vi "input.vi"(8 "error in":errorcluster, 10 "data table in":T5, 11 "SystemLin Tag Module runtime in":refnum<class "SystemLink runtime.lvclass">) -> (0 "error out":errorcluster, 2 "data table out":T5, 3 "SystemLin Tag Module runtime out":refnum<class "SystemLink runtime.lvclass">)   [LabVIEW 2015, in "SystemLink runtime.lvclass"]
doc: "Provides an interface for reading data from a module at runtime. While this interface performs no operations, a child should provide an override which may read from any open sessions, references, or interfaces."
uses:
  SystemLink runtime.lvclass
  <vilib>/NI/Tag Bus/table/data table.ctl
  <vilib>/Skyline/Tag/Shared/typedefs/Tag Value Cluster.ctl
  <vilib>/Skyline/Tag/Shared/typedefs/DataType.ctl
  configuration/SysLink Mapping.ctl
  <vilib>/Skyline/Tag/Wrapper/Wrapper_class/NI Skyline Tag.lvclass
  <vilib>/NI/Tag Bus/tag/Data Type.ctl
  SystemLink runtime.lvclass/SystemLink runtime.ctl
  <vilib>/NI/Tag Bus/table/data polymorphs/write one/write Double.vi
  <vilib>/NI/Tag Bus/table/data polymorphs/write one/write Single.vi
  <vilib>/NI/Tag Bus/table/data polymorphs/write one/write String.vi
  <vilib>/NI/Tag Bus/table/data polymorphs/write one/write I32.vi
  <vilib>/NI/Tag Bus/table/data polymorphs/write one/write U64.vi
  <vilib>/NI/Tag Bus/table/data polymorphs/write one/write I16.vi
  <vilib>/NI/Tag Bus/table/data polymorphs/write one/write I8.vi
  <vilib>/NI/Tag Bus/table/data polymorphs/write one/write Boolean.vi
  <vilib>/NI/Tag Bus/table/data table.lvlib
  <vilib>/Skyline/Tag/Wrapper/Wrapper_class/Read Tag (I32).vi
  <vilib>/Skyline/Tag/Wrapper/Wrapper_class/Read Tag (DBL).vi
  <vilib>/Skyline/Tag/Wrapper/Wrapper_class/Read Tag (String).vi
  <vilib>/Skyline/Tag/Shared/NI Skyline Tag.lvlib
  <vilib>/NI/Tag Bus/tag/tag descriptor.lvclass
  configuration/SystemLink configuration.lvclass
panel:
  out "Inputs Array":refnum<class "NI Skyline Tag.lvclass">[](array[class])
  out "Input Map":T1[](array[typedef])
  out "tag clusters":T3[](array[typedef])
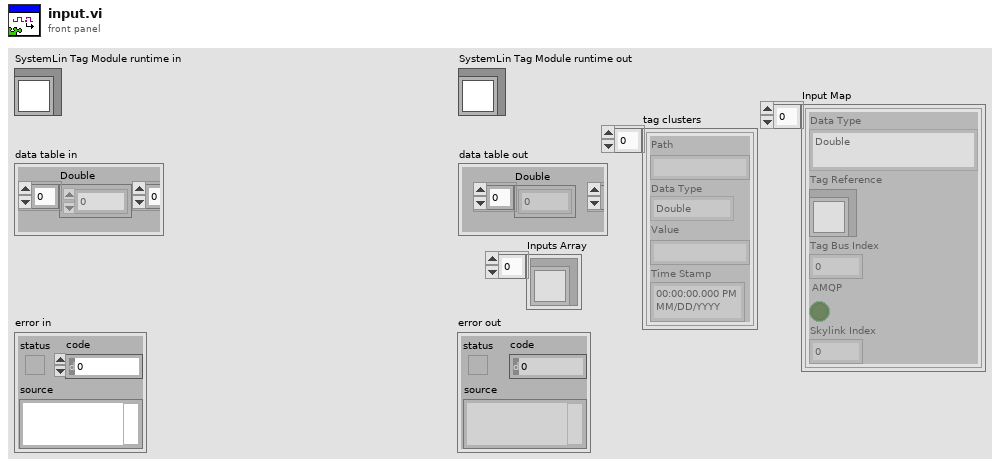
[diagram p1: front panel]
types:
  T1 = typedef "SystemLink configuration.lvclass/SysLink Mapping.ctl" = cluster{"Data Type":T2, "Tag Reference":refnum<class "NI Skyline Tag.lvclass">, "Tag Bus Index":i32, "AMQP":bool, "Skylink Index":i32}
  T2 = typedef "tag bus.lvlib/tag descriptor.lvclass/Data Type.ctl" = enum16{"Double", "Single", "I64", "I32", "I16", "I8", "U64", "U32", "U16", "U8", "Boolean", "String", "Array of Double", "Array of Single", "Array of I64", "Array of I32", "Array of I16", "Array of I8", "Array of U64", "Array of U32", "Array of U16", "Array of U8", "Array of Boolean", "Array of String"}
  T3 = typedef "NI Skyline Tag.lvlib/Tag Value Cluster.ctl" = cluster{"Path":string, "Data Type":T4, "Value":string, "Time Stamp":timestamp}
  T4 = typedef "NI Skyline Tag.lvlib/DataType.ctl" = enum32{"Double", "I32", "String", "Boolean", "U64", "Timestamp"}
  T5 = typedef "tag bus.lvlib/data table.lvlib/data table.ctl" = cluster{"Double":dbl[], "Single":sgl[], "I64":i64[], "I32":i32[], "I16":i16[], "I8":i8[], "U64":u64[], "U32":u32[], "U16":u16[], "U8":u8[], "Boolean":bool[], "String":string[], "Array of Double":cluster{"DBL Array":dbl[]}[], "Array of Single":cluster{"SGL Array":sgl[]}[], "Array of I64":cluster{"I64 Array":i64[]}[], "Array of I32":cluster{"I32 Array":i32[]}[], "Array of I16":cluster{"I16 Array":i16[]}[], "Array of I8":cluster{"I8 Array":i8[]}[], "Array of U64":cluster{"U64 Array":u64[]}[], "Array of U32":cluster{"U32 Array":u32[]}[], "Array of U16":cluster{"U16 Array":u16[]}[], "Array of U8":cluster{"U8 Array":u8[]}[], "Array of Boolean":cluster{"Boolean Array":bool[]}[], "Array of String":cluster{"String Array":string[]}[]}
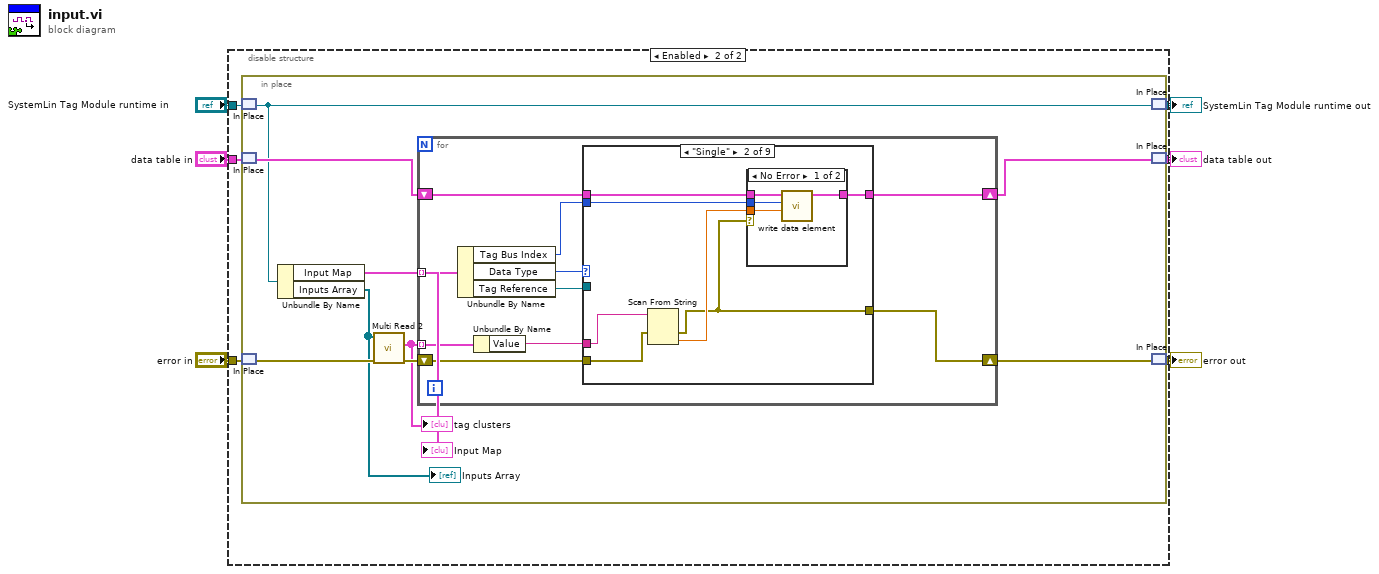
[diagram p0: block diagram]
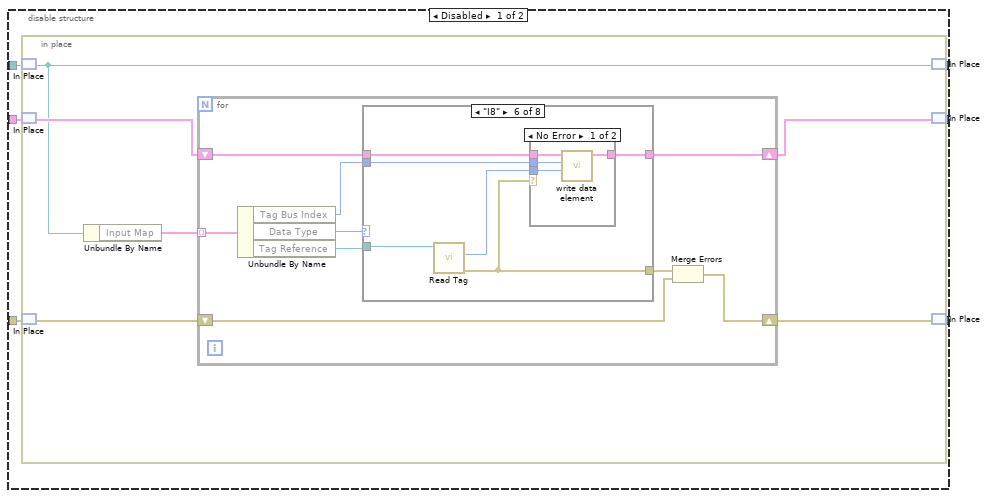
[diagram p2: hidden frame]
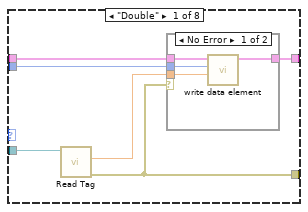
[diagram p3: hidden frame]
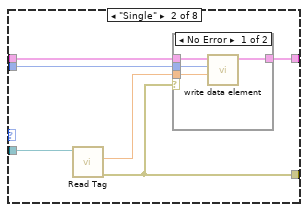
[diagram p5: hidden frame]
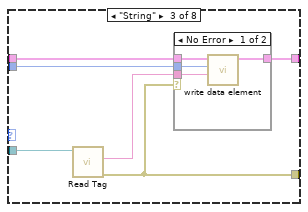
[diagram p7: hidden frame]
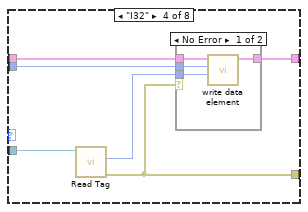
[diagram p9: hidden frame]
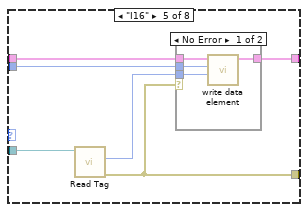
[diagram p11: hidden frame]
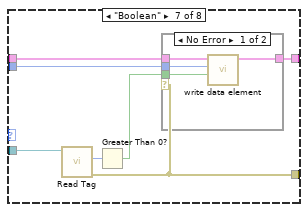
[diagram p14: hidden frame]
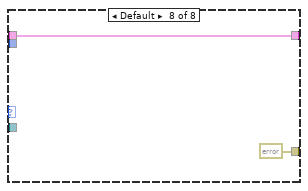
[diagram p16: hidden frame]
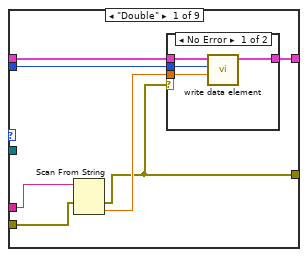
[diagram p17: hidden frame]
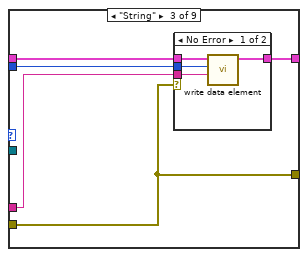
[diagram p20: hidden frame]
diagram:
  n1 = disable-structure shown="Enabled" {
    disable-tunnel: "SystemLin Tag Module runtime in" -> [w12 w113]
    disable-tunnel: [w11 w112] -> w5
    disable-tunnel: "data table in" -> [w10 w111]
    disable-tunnel: [w9 w110] -> w3
    disable-tunnel: [w8 w109] -> w2
    disable-tunnel: "error in" -> [w7 w108]
    frame Disabled {
      n2 = in-place {
        n3 = in-place-match #1(w12) -> (w14:refnum<class "SystemLink runtime.lvclass">)
        n4 = in-place-match #2(w10) -> (w18:T5)
        n5 = in-place-match #3(w7) -> (w16:errorcluster)
        n6 = Unbundle By Name(w14) -> ("Input Map"=w13:T1[])
        n7 = for {
          shift-right: [w24] -> w17
          shift-left: w18 -> [w25]
          shift-right: [w21] -> w15
          shift-left: w16 -> [w20]
          tunnel: w13 -> [w27] mode=indexing
          n8 = Unbundle By Name(w27) -> ("Tag Bus Index"=w23:i32, "Data Type"=w26:T2, "Tag Reference"=w19:refnum<class "NI Skyline Tag.lvclass">)
          n9 = case shown="\"I8\"" w26 {
            tunnel: w25 -> [w33 w44 w55 w66 w77 w88 w100 w107]
            tunnel: [w32 w43 w54 w65 w76 w87 w99 w107] -> w24
            tunnel: w23 -> [w31 w42 w53 w64 w75 w86 w98 _]
            tunnel: w19 -> [w30 w41 w52 w63 w74 w85 w97 _]
            tunnel: [w28 w39 w50 w61 w72 w83 w96 errorcluster {"status"=FALSE, "code"=0, "source"=""} ("error IO")] -> w22
            frame "Double" {
              n10 = call-poly <vilib>:"Read Tag.vi"("tag in"=w30) -> ("error out"=w28:errorcluster, "value"=w29:dbl)  [unwired: 6 in, 3 out]
              n11 = case shown="No Error" w28 {
                tunnel: w33 -> [w37 w38]
                tunnel: [w36 w38] -> w32
                tunnel: w31 -> [w35 _]
                tunnel: w29 -> [w34 _]
                frame No Error {
                  n12 = call-poly <vilib>:"write data element.vi"("value"=w34, "index"=w35, "data table in"=w37) -> ("data table out"=w36:T5)  [unwired: 8 in]
                }
                frame Error {
                }
              }
            }
            frame "Single" {
              n13 = call-poly <vilib>:"Read Tag.vi"("tag in"=w41) -> ("error out"=w39:errorcluster, "value"=w40:dbl)  [unwired: 6 in, 3 out]
              n14 = case shown="No Error" w39 {
                tunnel: w44 -> [w48 w49]
                tunnel: [w47 w49] -> w43
                tunnel: w42 -> [w46 _]
                tunnel: w40 -> [w45 _]
                frame No Error {
                  n15 = call-poly <vilib>:"write data element.vi"("value"=w45, "index"=w46, "data table in"=w48) -> ("data table out"=w47:T5)  [unwired: 8 in]
                }
                frame Error {
                }
              }
            }
            frame "String" {
              n16 = call-poly <vilib>:"Read Tag.vi"("tag in"=w52) -> ("error out"=w50:errorcluster, "value"=w51:string)  [unwired: 6 in, 3 out]
              n17 = case shown="No Error" w50 {
                tunnel: w55 -> [w59 w60]
                tunnel: [w58 w60] -> w54
                tunnel: w53 -> [w57 _]
                tunnel: w51 -> [w56 _]
                frame No Error {
                  n18 = call-poly <vilib>:"write data element.vi"("value"=w56, "index"=w57, "data table in"=w59) -> ("data table out"=w58:T5)  [unwired: 8 in]
                }
                frame Error {
                }
              }
            }
            frame "I32" {
              n19 = call-poly <vilib>:"Read Tag.vi"("tag in"=w63) -> ("error out"=w61:errorcluster, "value"=w62:i32)  [unwired: 6 in, 3 out]
              n20 = case shown="No Error" w61 {
                tunnel: w66 -> [w70 w71]
                tunnel: [w69 w71] -> w65
                tunnel: w64 -> [w68 _]
                tunnel: w62 -> [w67 _]
                frame No Error {
                  n21 = call-poly <vilib>:"write data element.vi"("value"=w67, "index"=w68, "data table in"=w70) -> ("data table out"=w69:T5)  [unwired: 8 in]
                }
                frame Error {
                }
              }
            }
            frame "I16" {
              n22 = call-poly <vilib>:"Read Tag.vi"("tag in"=w74) -> ("error out"=w72:errorcluster, "value"=w73:i32)  [unwired: 6 in, 3 out]
              n23 = case shown="No Error" w72 {
                tunnel: w77 -> [w81 w82]
                tunnel: [w80 w82] -> w76
                tunnel: w75 -> [w79 _]
                tunnel: w73 -> [w78 _]
                frame No Error {
                  n24 = call-poly <vilib>:"write data element.vi"("value"=w78, "index"=w79, "data table in"=w81) -> ("data table out"=w80:T5)  [unwired: 8 in]
                }
                frame Error {
                }
              }
            }
            frame "I8" {
              n25 = call-poly <vilib>:"Read Tag.vi"("tag in"=w85) -> ("error out"=w83:errorcluster, "value"=w84:i32)  [unwired: 6 in, 3 out]
              n26 = case shown="No Error" w83 {
                tunnel: w88 -> [w92 w93]
                tunnel: [w91 w93] -> w87
                tunnel: w86 -> [w90 _]
                tunnel: w84 -> [w89 _]
                frame No Error {
                  n27 = call-poly <vilib>:"write data element.vi"("value"=w89, "index"=w90, "data table in"=w92) -> ("data table out"=w91:T5)  [unwired: 8 in]
                }
                frame Error {
                }
              }
            }
            frame "Boolean" {
              n28 = call-poly <vilib>:"Read Tag.vi"("tag in"=w97) -> ("error out"=w96:errorcluster, "value"=w95:i32)  [unwired: 6 in, 3 out]
              n29 = Greater Than 0?(x=w95) -> (x > 0?=w94:bool)
              n30 = case shown="No Error" w96 {
                tunnel: w100 -> [w104 w105]
                tunnel: [w103 w105] -> w99
                tunnel: w98 -> [w102 _]
                tunnel: w94 -> [w101 _]
                frame No Error {
                  n31 = call-poly <vilib>:"write data element.vi"("value"=w101, "index"=w102, "data table in"=w104) -> ("data table out"=w103:T5)  [unwired: 8 in]
                }
                frame Error {
                }
              }
            }
            frame Default {
            }
          }
          n32 = Merge Errors(w22, w20) -> (w21:errorcluster)
        }
        n33 = in-place-match #1(w14) -> (w11:refnum<class "SystemLink runtime.lvclass">)
        n34 = in-place-match #2(w17) -> (w9:T5)
        n35 = in-place-match #3(w15) -> (w8:errorcluster)
      }
    }
    frame Enabled {
      n36 = in-place {
        n37 = in-place-match #4(w113) -> (w119:refnum<class "SystemLink runtime.lvclass">)
        n38 = in-place-match #5(w111) -> (w122:T5)
        n39 = in-place-match #6(w108) -> (w117:errorcluster)
        n40 = Unbundle By Name(w119) -> ("Input Map"=w118:T1[], "Inputs Array"=w115:refnum<class "NI Skyline Tag.lvclass">[])
        "Input Map" <- w118
        "Inputs Array" <- w115
        n41 = call <vilib>:"Multi Read 2.vi"("error in (no error)"=w117, "tags in"=w115) -> ("error out"=w116:errorcluster, "tag clusters"=w114:T3[])  [unwired: 7 in, 1 out]
        "tag clusters" <- w114
        n42 = for {
          shift-right: [w129] -> w121
          shift-left: w122 -> [w130]
          shift-right: [w127] -> w120
          shift-left: w116 -> [w123]
          tunnel: w118 -> [w132] mode=indexing
          tunnel: w114 -> [w125] mode=indexing
          n43 = Unbundle By Name(w132) -> ("Tag Bus Index"=w128:i32, "Data Type"=w131:T2, "Tag Reference"=w126:refnum<class "NI Skyline Tag.lvclass">)
          n44 = Unbundle By Name(w125) -> ("Value"=w124:string)
          n45 = case shown="\"Single\"" w131 {
            tunnel: w130 -> [w139 w151 w161 w174 w187 w200 w213 w225 w232]
            tunnel: [w138 w150 w160 w173 w186 w199 w212 w224 w232] -> w129
            tunnel: w128 -> [w137 w149 w159 w172 w185 w198 w211 w223 _]
            tunnel: w126 -> [_ _ _ _ _ _ _ _ _]
            tunnel: [w133 w145 w157 w168 w182 w193 w208 w219 errorcluster {"status"=FALSE, "code"=0, "source"=""} ("error IO")] -> w127
            tunnel: w124 -> [w136 w148 w158 w170 w184 w197 w210 w222 _]
            tunnel: w123 -> [w135 w147 w157 w169 w183 w196 w209 w219 _]
            frame "Double" {
              n46 = Scan From String(input string=w136, error in=w135) -> (error out=w133:errorcluster, output 1=w134:dbl)  [unwired: 3 in, 2 out]
              n47 = case shown="No Error" w133 {
                tunnel: w139 -> [w143 w144]
                tunnel: [w142 w144] -> w138
                tunnel: w137 -> [w141 _]
                tunnel: w134 -> [w140 _]
                frame No Error {
                  n48 = call-poly <vilib>:"write data element.vi"("value"=w140, "index"=w141, "data table in"=w143) -> ("data table out"=w142:T5)  [unwired: 8 in]
                }
                frame Error {
                }
              }
            }
            frame "Single" {
              n49 = Scan From String(input string=w148, error in=w147) -> (error out=w145:errorcluster, output 1=w146:dbl)  [unwired: 3 in, 2 out]
              n50 = case shown="No Error" w145 {
                tunnel: w151 -> [w155 w156]
                tunnel: [w154 w156] -> w150
                tunnel: w149 -> [w153 _]
                tunnel: w146 -> [w152 _]
                frame No Error {
                  n51 = call-poly <vilib>:"write data element.vi"("value"=w152, "index"=w153, "data table in"=w155) -> ("data table out"=w154:T5)  [unwired: 8 in]
                }
                frame Error {
                }
              }
            }
            frame "String" {
              n52 = case shown="No Error" w157 {
                tunnel: w161 -> [w165 w166]
                tunnel: [w164 w166] -> w160
                tunnel: w159 -> [w163 _]
                tunnel: w158 -> [w162 _]
                frame No Error {
                  n53 = call-poly <vilib>:"write data element.vi"("value"=w162, "index"=w163, "data table in"=w165) -> ("data table out"=w164:T5)  [unwired: 8 in]
                }
                frame Error {
                }
              }
            }
            frame "I32" {
              n54 = Scan From String(input string=w170, error in=w169, default 1=0 ("value")) -> (error out=w168:errorcluster, output 1=w167:i32)  [unwired: 2 in, 2 out]
              n55 = case shown="No Error" w168 {
                tunnel: w174 -> [w178 w179]
                tunnel: [w177 w179] -> w173
                tunnel: w172 -> [w176 _]
                tunnel: w167 -> [w175 _]
                frame No Error {
                  n56 = call-poly <vilib>:"write data element.vi"("value"=w175, "index"=w176, "data table in"=w178) -> ("data table out"=w177:T5)  [unwired: 8 in]
                }
                frame Error {
                }
              }
            }
            frame "U64" {
              n57 = Scan From String(input string=w184, error in=w183, default 1=u64 0 ("value")) -> (error out=w182:errorcluster, output 1=w181:u64)  [unwired: 2 in, 2 out]
              n58 = case shown="No Error" w182 {
                tunnel: w187 -> [w191 w192]
                tunnel: [w190 w192] -> w186
                tunnel: w185 -> [w189 _]
                tunnel: w181 -> [w188 _]
                frame No Error {
                  n59 = call-poly <vilib>:"write data element.vi"("value"=w188, "index"=w189, "data table in"=w191) -> ("data table out"=w190:T5)  [unwired: 8 in]
                }
                frame Error {
                }
              }
            }
            frame "I16" {
              n60 = Scan From String(input string=w197, error in=w196, default 1=i16 0 ("value")) -> (error out=w193:errorcluster, output 1=w195:i16)  [unwired: 2 in, 2 out]
              n61 = case shown="No Error" w193 {
                tunnel: w200 -> [w204 w205]
                tunnel: [w203 w205] -> w199
                tunnel: w198 -> [w202 _]
                tunnel: w195 -> [w201 _]
                frame No Error {
                  n62 = call-poly <vilib>:"write data element.vi"("value"=w201, "index"=w202, "data table in"=w204) -> ("data table out"=w203:T5)  [unwired: 8 in]
                }
                frame Error {
                }
              }
            }
            frame "I8" {
              n63 = Scan From String(input string=w210, error in=w209, default 1=i8 0 ("value")) -> (error out=w208:errorcluster, output 1=w207:i8)  [unwired: 2 in, 2 out]
              n64 = case shown="No Error" w208 {
                tunnel: w213 -> [w217 w218]
                tunnel: [w216 w218] -> w212
                tunnel: w211 -> [w215 _]
                tunnel: w207 -> [w214 _]
                frame No Error {
                  n65 = call-poly <vilib>:"write data element.vi"("value"=w214, "index"=w215, "data table in"=w217) -> ("data table out"=w216:T5)  [unwired: 8 in]
                }
                frame Error {
                }
              }
            }
            frame "Boolean" {
              n66 = Equal?(x="True", y=w222) -> (x = y?=w220:bool)
              n67 = case shown="No Error" w219 {
                tunnel: w225 -> [w229 w230]
                tunnel: [w228 w230] -> w224
                tunnel: w223 -> [w227 _]
                tunnel: w220 -> [w226 _]
                frame No Error {
                  n68 = call-poly <vilib>:"write data element.vi"("value"=w226, "index"=w227, "data table in"=w229) -> ("data table out"=w228:T5)  [unwired: 8 in]
                }
                frame Error {
                }
              }
            }
            frame Default {
            }
          }
        }
        n69 = in-place-match #4(w119) -> (w112:refnum<class "SystemLink runtime.lvclass">)
        n70 = in-place-match #5(w121) -> (w110:T5)
        n71 = in-place-match #6(w120) -> (w109:errorcluster)
      }
    }
  }
  "error out" <- w2
  "SystemLin Tag Module runtime out" <- w5
  "data table out" <- w3
